vi "comunicaçaoserial(read0.vi"() -> ()   [LabVIEW 2024]
uses:
  <vilib>/Instr/_visa.llb/VISA Configure Serial Port (Instr).vi
panel:
  out "Waveform Chart 2":dbl(graph)
  out "output 2":dbl
  out "Waveform Chart":dbl(graph)
  out "output 1":dbl
  in  "termination char\n(0xA = '\\n' = LF)":u8=10 format="%.0x"
  out "read buffer":string
  in  "operation":dbl
  in  "VISA resource name":refnum<visa-resource-name>
  in  "String":string
  in  "stop":bool
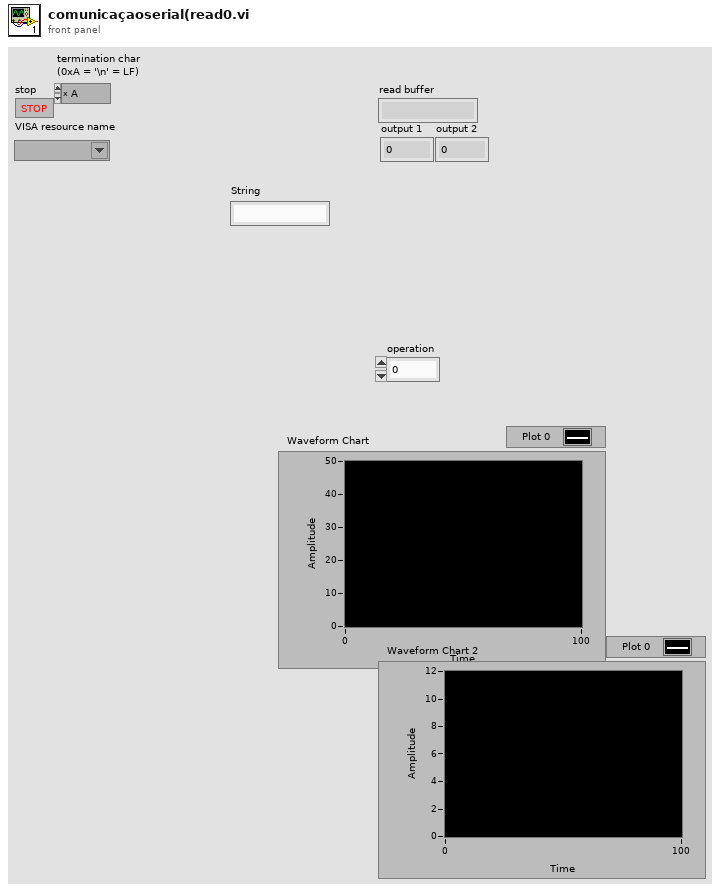
[diagram p1: front panel]
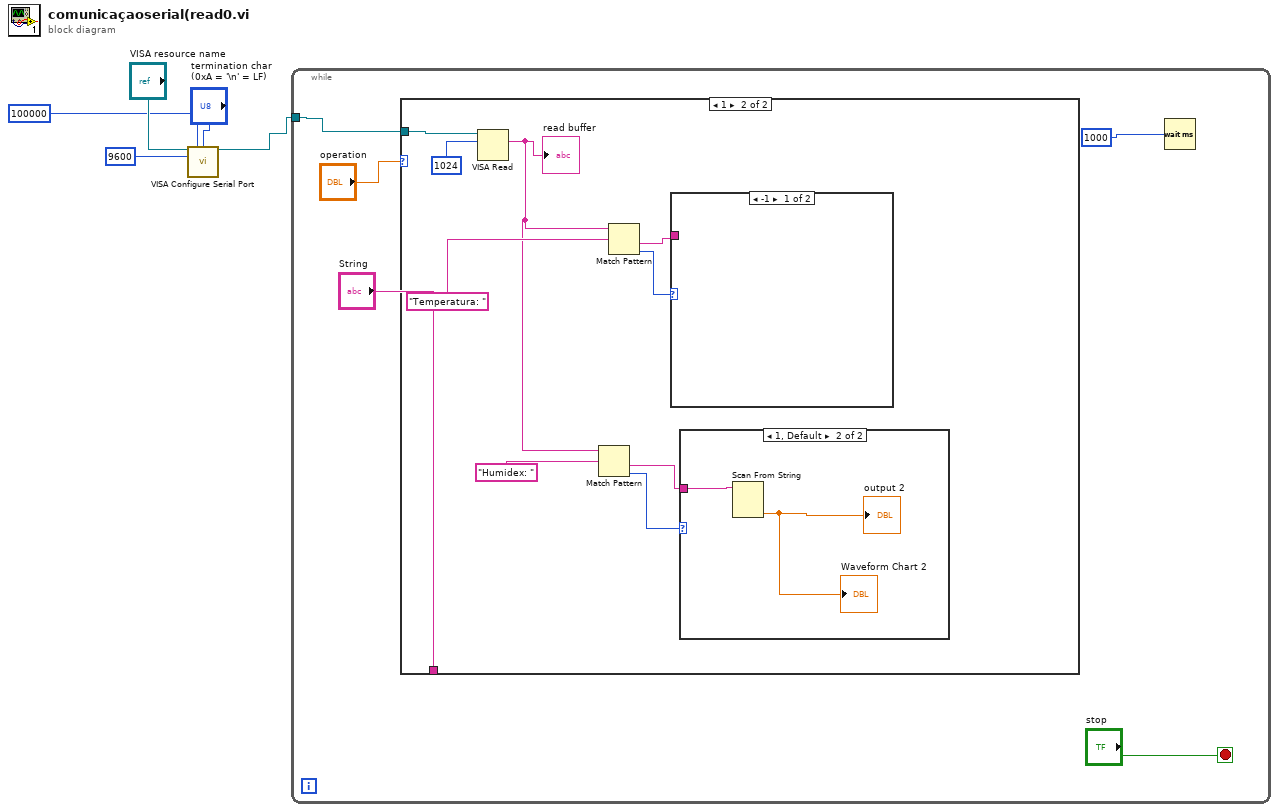
[diagram p0: block diagram]
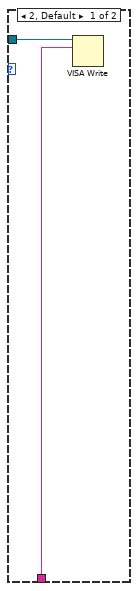
[diagram p2: hidden frame]
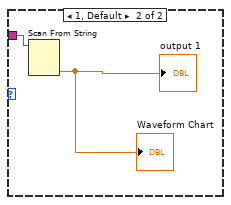
[diagram p4: hidden frame]
diagram:
  n1 = call-poly "VISA Configure Serial Port"("VISA resource name"="VISA resource name", "timeout (10sec)"=u32 100000, "termination char\n(0xA = '\\n' = LF)"="termination char\n(0xA = '\\n' = LF)", "baud rate (9600)"=u32 9600) -> ("VISA resource name out"=w4:refnum<visa-resource-name>)  [unwired: 10 in, 1 out]
  n2 = while {
    tunnel: w4 -> [w9]
    stop <- "stop" stop-if-true
    n3 = case shown="1" "operation" {
      tunnel: w9 -> [w12 w21]
      tunnel: "String" -> [w11 _]
      frame 2, Default {
        n4 = VISA Write(VISA resource name=w12, write buffer=w11) -> ()  [unwired: 1 in, 3 out]
      }
      frame 1 {
        n5 = VISA Read(VISA resource name=w21, byte count=u32 1024) -> (read buffer=w17:string)  [unwired: 1 in, 3 out]
        "read buffer" <- w17
        n6 = Match Pattern(string=w17, regular expression="Humidex: ") -> (after substring=w13:string, offset past match=w15:i32)  [unwired: 1 in, 2 out]
        n7 = Match Pattern(string=w17, regular expression="Temperatura: ") -> (after substring=w14:string, offset past match=w16:i32)  [unwired: 1 in, 2 out]
        n8 = case shown="-1" w16 {
          tunnel: w14 -> [_ w25]
          frame -1 {
          }
          frame 1, Default {
            n9 = Scan From String(input string=w25) -> (output 1=→"output 1" →"Waveform Chart":dbl)  [unwired: 4 in, 3 out]
          }
        }
        n10 = case shown="1, Default" w15 {
          tunnel: w13 -> [_ w22]
          frame -1 {
          }
          frame 1, Default {
            n11 = Scan From String(input string=w22) -> (output 1=→"output 2" →"Waveform Chart 2":dbl)  [unwired: 4 in, 3 out]
          }
        }
      }
    }
    n12 = Wait (ms)(milliseconds to wait=u32 1000) -> ()  [unwired: 1 out]
  }
